vi "Read Attributes.vi"(11 "Shutdown Microgrid Msg":refnum<class "Shutdown Microgrid Msg.lvclass">) -> (2 "Payload":cluster{"Data":variant})   [LabVIEW 2018, in "Remote Operation Abstract.lvlib" / "Shutdown Microgrid Msg.lvclass"]
uses:
  Shutdown Microgrid Msg.lvclass
  Shutdown Microgrid Msg.lvclass/Shutdown Microgrid Msg.ctl
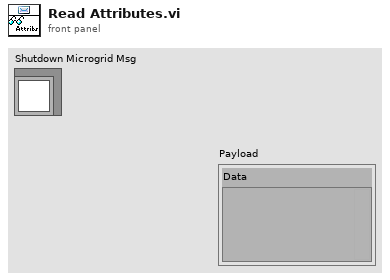
[diagram p1: front panel]
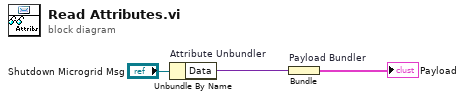
[diagram p0: block diagram]
diagram:
  n1 = Unbundle By Name "Attribute Unbundler"("Shutdown Microgrid Msg") -> ("Data"=w1:variant)
  n2 = Bundle "Payload Bundler"("Data"=w1) -> (→"Payload":cluster{"Data":variant})  [unwired: 1 in]
